vi "Config AO DC.vi"(6 "Channel config":T1={"Voltage"=1.0, "physical channels"="", "name to assign"=""}, 8 "error in":errorcluster, 11 "task in":refnum<k21>) -> (0 "error out":errorcluster, 3 "task out":refnum<k21>)   [LabVIEW 2019]
doc: "This example demonstrates how to acquire a continuous amount of data (Waveform) using the DAQ device's internal clock. It also shows how to synchronize two devices for different device families (E Series, S Series, M Series, X Series, DSA, and SC Express), to simultaneously acquire the data.\n\nFor instructions on how to connect your signals to the DAQ device, refer to your device documentation."
uses:
  <vilib>/DAQmx/create/channels.llb/DAQmx Create Channel (AO-Voltage-Basic).vi
  <vilib>/DAQmx/miscellaneous.llb/DAQmx Fill In Error Info.vi
  <vilib>/DAQmx/write.llb/DAQmx Write (Analog DBL 1Chan 1Samp).vi
panel:
  # "Config AO - DC"
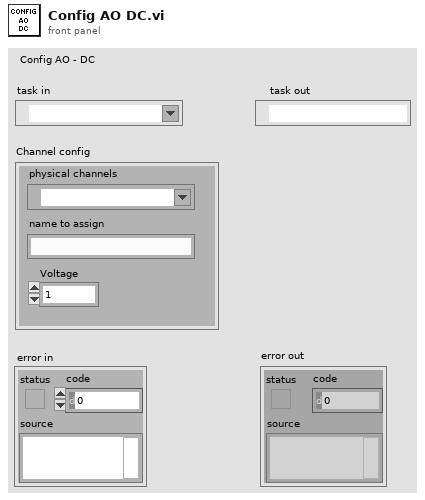
[diagram p1: front panel]
types:
  T1 = cluster{"Voltage":dbl, "physical channels":tag, "name to assign":string}
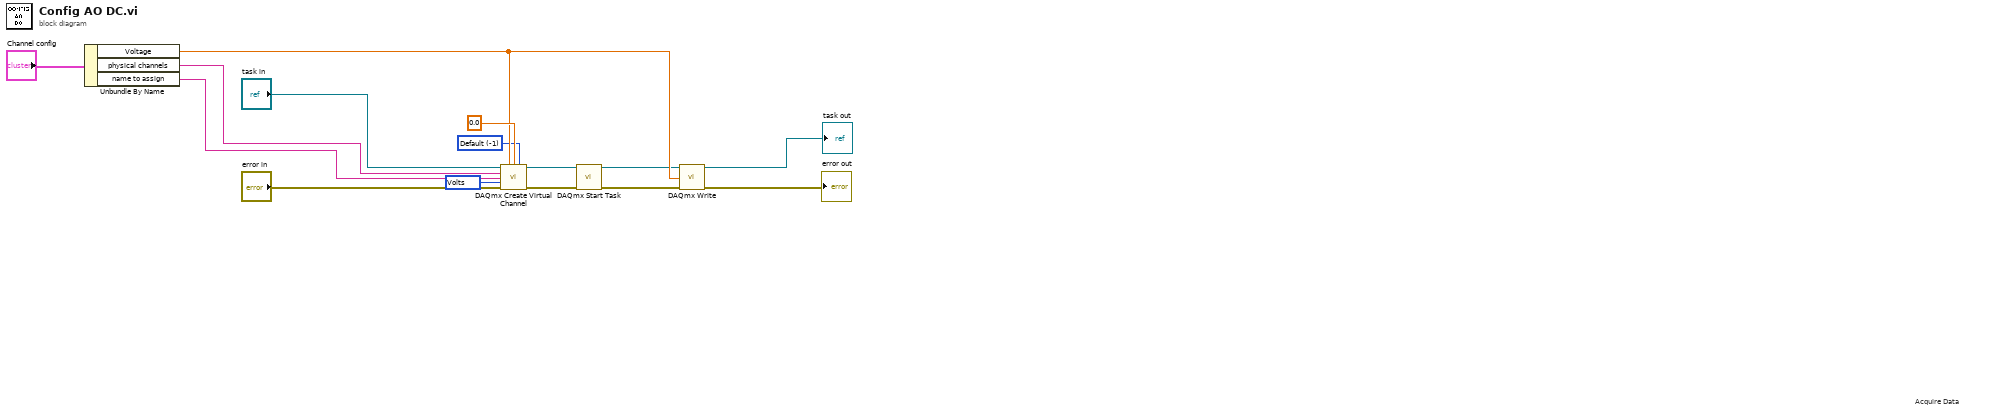
[diagram p0: block diagram]
diagram:
  w5 = 10348 items=["Volts"=10348, "From Custom Scale"=10065] ("units")
  w6 = -1 items=["Default"=-1, "RSE"=10083, "Differential"=10106, "Pseudodifferential"=12529] ("output terminal configuration")
  # "Acquire Data"
  n1 = Unbundle By Name("Channel config") -> ("Voltage"=w7:dbl, "physical channels"=w9:tag, "name to assign"=w8:string)
  n2 = call-poly <vilib>:"DAQmx Create Virtual Channel.vi"("task in"="task in", "maximum value"=w7, "minimum value"=0.0, "output terminal configuration"=w6, "physical channels"=w9, "name to assign"=w8, "units"=w5, "error in"="error in") -> ("task out"=w4:refnum<k21>, "error out"=w2:errorcluster)  [unwired: 6 in]
  n3 = call <vilib>:"DAQmx Start Task.vi"("task/channels in"=w4, "error in"=w2) -> ("task out"=w3:refnum<k21>, "error out"=w1:errorcluster)  [unwired: 12 in]
  n4 = call-poly <vilib>:"DAQmx Write.vi"("task/channels in"=w3, "data"=w7, "error in"=w1) -> ("task out"=→"task out":refnum<k21>, "error out"=→"error out":errorcluster)  [unwired: 10 in, 1 out]
